vi "repeat cycle.vi"(8 "error in (no error)":errorcluster caption="에러 입력(에러 없음)", 10 "waveform":waveform(dbl), 11 "Waveform Obj 입력":refnum<class "Waveform Gen.lvclass">) -> (0 "error out":errorcluster caption="에러 출력", 2 "waveform out":waveform(dbl), 3 "Waveform Obj 출력":refnum<class "Waveform Gen.lvclass">)   [LabVIEW 2020, in "Waveform Gen.lvclass"]
uses:
  Waveform Gen.lvclass
  Waveform Gen.lvclass/Waveform Gen.ctl
  Accessors/Read repeat type.vi
  <vilib>/Waveform/WDTOps.llb/WDT Append Waveforms DBL.vi
  <vilib>/Waveform/WDTOps.llb/WDT Get Waveform Subset DBL.vi
  <vilib>/Waveform/WDTOps.llb/WDT Number of Waveform Samples DBL.vi
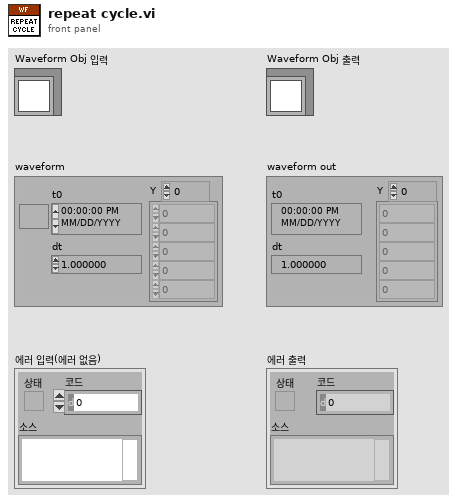
[diagram p1: front panel]
types:
  T1 = typedef "Waveform Gen.lvclass/repeat scale.ctl" = enum16{"Normal", "Lin. Up", "Lin. Down", "Exp. Up", "Exp. Down"}
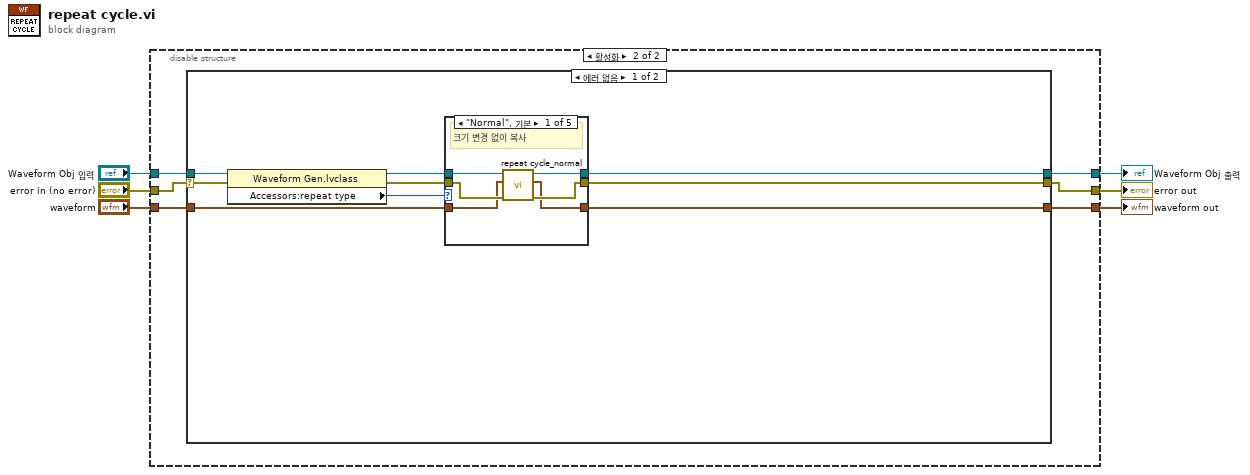
[diagram p0: block diagram]
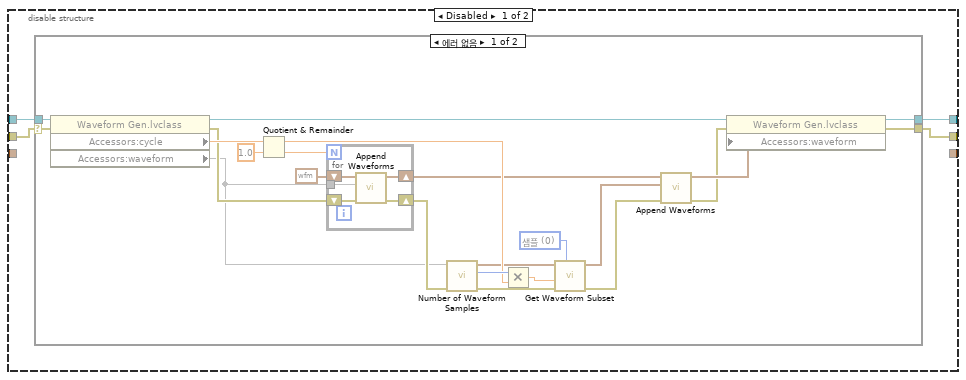
[diagram p2: hidden frame]
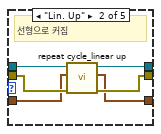
[diagram p4: hidden frame]
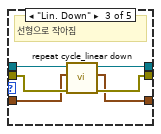
[diagram p5: hidden frame]
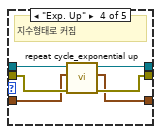
[diagram p6: hidden frame]
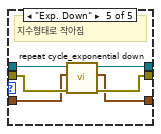
[diagram p7: hidden frame]
diagram:
  n1 = disable-structure shown="활성화" {
    disable-tunnel: "Waveform Obj 입력" -> [w10 w45]
    disable-tunnel: [w9 w44] -> w5
    disable-tunnel: [w8 w43] -> w4
    disable-tunnel: "error in (no error)" -> [w7 w46]
    disable-tunnel: "waveform" -> [_ w42]
    disable-tunnel: [_ w41] -> w1
    frame Disabled {
      n2 = case shown="에러 없음" w7 {
        selector: w7 -> [w29 w40]
        tunnel: [w21 w40] -> w8
        tunnel: w10 -> [w33 w39]
        tunnel: [w23 w39] -> w9
        frame No Error {
          w15 = u16 0 items=["샘플", "상대 시간"] ("start/duration format")
          n3 = property class="Waveform Gen.lvclass"(reference=w33, error in=w29) -> (reference out=w32:refnum<class "Waveform Gen.lvclass">, error out=w19:errorcluster, "Accessors:cycle"=w31:dbl, "Accessors:waveform"=w13)
          n4 = Quotient & Remainder(x=w31, y=1.0) -> (x-y*floor(x/y)=w26:dbl, floor(x/y)=w28:dbl)
          n5 = for {
            N: w28 -> [_]
            shift-right: [w37] -> w12
            shift-left: waveform(dbl) {"t0"=timestamp(0 s since 1904-01-01), "dt"=1.0, "Y"=[]} ("waveform out") -> [w38]
            shift-right: [w35] -> w18
            shift-left: w19 -> [w36]
            tunnel: w13 -> [w34]
            n6 = call-poly <vilib>:"Append Waveforms.vi"("error in (no error)"=w36, "waveform B"=w34, "waveform A"=w38) -> ("error out"=w35:errorcluster, "waveform out"=w37:waveform(dbl))  [unwired: 7 in]
          }
          n7 = call-poly <vilib>:"Number of Waveform Samples.vi"("error in (no error)"=w18, "waveform in"=w13) -> ("error out"=w24:errorcluster, "number of samples"=w27:i32, "waveform out"=w16:waveform(dbl))  [unwired: 7 in]
          n8 = Multiply(x=w27, y=w26) -> (x*y=w25:dbl)
          n9 = call-poly <vilib>:"Get Waveform Subset.vi"("start/duration format"=w15, "error in (no error)"=w24, "duration"=w25, "waveform in"=w16) -> ("error out"=w17:errorcluster, "waveform out"=w11:waveform(dbl))  [unwired: 2 in, 2 out]
          n10 = call-poly <vilib>:"Append Waveforms.vi"("error in (no error)"=w17, "waveform B"=w11, "waveform A"=w12) -> ("error out"=w14:errorcluster, "waveform out"=w22:waveform(dbl))  [unwired: 7 in]
          n11 = property class="Waveform Gen.lvclass"(reference=w32, error in=w14, "Accessors:waveform"=w22) -> (reference out=w23:refnum<class "Waveform Gen.lvclass">, error out=w21:errorcluster)
        }
        frame Error {
        }
      }
    }
    frame Enabled {
      n12 = case shown="에러 없음" w46 {
        selector: w46 -> [w54 w86]
        tunnel: w45 -> [w55 w87]
        tunnel: [w49 w87] -> w44
        tunnel: [w50 w86] -> w43
        tunnel: w42 -> [w48 _]
        tunnel: [w47 _] -> w41
        frame No Error {
          n13 = property class="Waveform Gen.lvclass"(reference=w55, error in=w54) -> (reference out=w52:refnum<class "Waveform Gen.lvclass">, error out=w51:errorcluster, "Accessors:repeat type"=w53:T1)
          n14 = case shown="\"Normal\", 기본" w53 {
            tunnel: w52 -> [w61 w67 w73 w79 w85]
            tunnel: w51 -> [w60 w66 w72 w78 w84]
            tunnel: [w59 w65 w71 w77 w83] -> w49
            tunnel: [w58 w64 w70 w76 w82] -> w50
            tunnel: w48 -> [w57 w63 w69 w75 w81]
            tunnel: [w56 w62 w68 w74 w80] -> w47
            frame "Normal", Default {
              # "크기 변경 없이 복사"
              n15 = call-dynamic "repeat cycle_normal.vi"("error in (no error)"=w60, "waveform in"=w57, "Waveform Obj 입력"=w61) -> ("error out"=w58:errorcluster, "waveform out"=w56:waveform(dbl), "Waveform Obj 출력"=w59:refnum<class "Waveform Gen.lvclass">)  [unwired: 6 in]
            }
            frame "Lin. Up" {
              # "선형으로 커짐"
              n16 = call-dynamic "repeat cycle_linear up.vi"("error in (no error)"=w66, "waveform in"=w63, "Waveform Obj 입력"=w67) -> ("error out"=w64:errorcluster, "waveform out"=w62:waveform(dbl), "Waveform Obj 출력"=w65:refnum<class "Waveform Gen.lvclass">)  [unwired: 6 in]
            }
            frame "Lin. Down" {
              # "선형으로 작아짐"
              n17 = call-dynamic "repeat cycle_linear down.vi"("error in (no error)"=w72, "waveform in"=w69, "Waveform Obj 입력"=w73) -> ("error out"=w70:errorcluster, "waveform out"=w68:waveform(dbl), "Waveform Obj 출력"=w71:refnum<class "Waveform Gen.lvclass">)  [unwired: 6 in]
            }
            frame "Exp. Up" {
              # "지수형태로 커짐"
              n18 = call-dynamic "repeat cycle_exponential up.vi"("error in (no error)"=w78, "waveform in"=w75, "Waveform Obj 입력"=w79) -> ("error out"=w76:errorcluster, "waveform out"=w74:waveform(dbl), "Waveform Obj 출력"=w77:refnum<class "Waveform Gen.lvclass">)  [unwired: 6 in]
            }
            frame "Exp. Down" {
              # "지수형태로 작아짐"
              n19 = call-dynamic "repeat cycle_exponential down.vi"("error in (no error)"=w84, "waveform in"=w81, "Waveform Obj 입력"=w85) -> ("error out"=w82:errorcluster, "waveform out"=w80:waveform(dbl), "Waveform Obj 출력"=w83:refnum<class "Waveform Gen.lvclass">)  [unwired: 6 in]
            }
          }
        }
        frame Error {
        }
      }
    }
  }
  "error out" <- w4
  "Waveform Obj 출력" <- w5
  "waveform out" <- w1
